vi "TriggerExample.vi"() -> ()   [LabVIEW 2016]
uses:
  controls/RunMode.ctl
  controls/TriggerNo.ctl
panel:
  out "Numeric":i32
  out "Message":string
  out "data out 2":string
  out "ExecConNo":i32
  out "RegisteredString":string
  out "ProgramNumber":i32
  out "SDCard":u16
  out "RunMode":T1
  out "error out":errorcluster
  out "data out":string
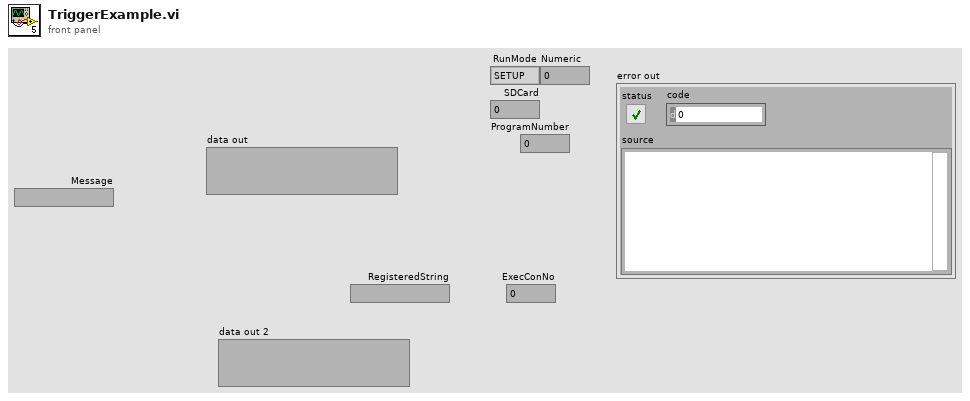
[diagram p1: front panel]
types:
  T1 = typedef "RunMode.ctl" = enum16{"SETUP", "RUN"}
  T2 = enum16{"Standard", "Buffered", "CRLF", "Immediate"}
  T3 = typedef "TriggerNo.ctl" = u8
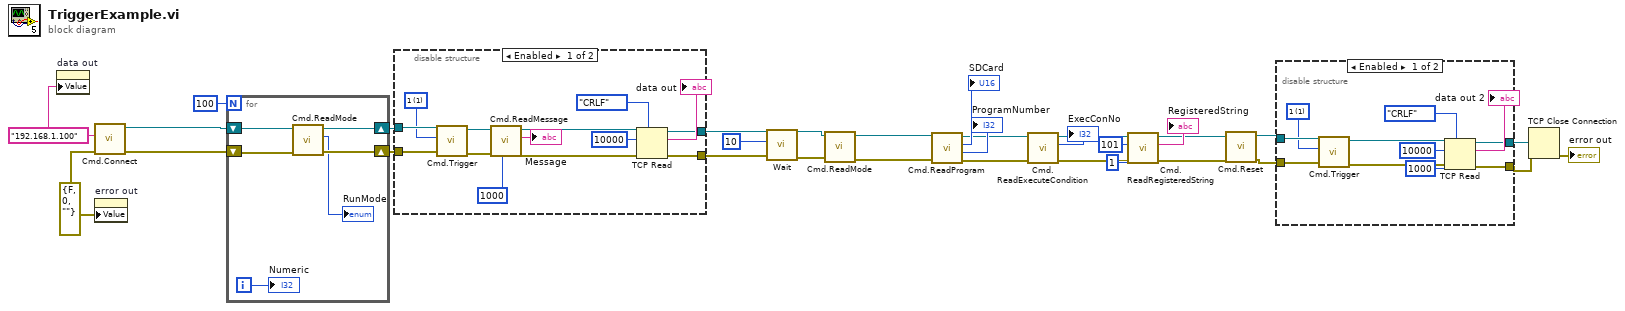
[diagram p0: block diagram]
diagram:
  w22 = errorcluster {"status"=FALSE, "code"=0, "source"=""} ("error constant")
  w21 = "192.168.1.100"
  n1 = property on="data out" class="Str"("Value"=w21) -> ()  [unwired: 2 in, 2 out]
  n2 = call "Cmd.Connect.vi"("error in (no error)"=w22, "IP"=w21) -> ("error out"=w2:errorcluster, "connection ID out"=w5:refnum<k5>)  [unwired: 8 in]
  n3 = property on="error out" class="Clust (strict)"("Value"=w22) -> ()  [unwired: 2 in, 2 out]
  n4 = for {
    N: 100 -> [_]
    shift-right: [w35] -> w4
    shift-left: w5 -> [w36]
    shift-right: [w34] -> w3
    shift-left: w2 -> [w33]
    i -> [w31]
    n5 = call "Cmd.ReadMode.vi"("error in"=w33, "cID in"=w36) -> ("error out"=w34:errorcluster, "RunMode"=→"RunMode":T1, "cID out"=w35:refnum<k5>)  [unwired: 7 in]
    "Numeric" <- w31
  }
  n6 = disable-structure shown="Enabled" {
    disable-tunnel: w4 -> [w50 w51]
    disable-tunnel: w3 -> [w49 w52]
    disable-tunnel: [w45 w52] -> w20
    disable-tunnel: [w44 w51] -> w17
    frame Enabled {
      w43 = T3 1 items=["1"=1, "2"=2, "3"=3, "4"=4, "ALL"=5] ("TriggerNo")
      n7 = call "Cmd.Trigger.vi"("error in"=w49, "TriggerNo"=w43, "cID in"=w50) -> ("error out"=w41:errorcluster, "cID out"=w42:refnum<k5>)  [unwired: 6 in, 1 out]
      n8 = call "Cmd.ReadMessage.vi"("Timeout [ms] (1000)"=1000 ("timeout ms (25000)"), "error in"=w41, "cID in"=w42) -> ("error out"=w39:errorcluster, "Message"=→"Message":string, "cID out"=w40:refnum<k5>)  [unwired: 6 in]
      n9 = TCP Read(connection ID=w40, bytes to read=10000, error in (no error)=w39, 7:T2."CRLF" ("mode (standard)")) -> (connection ID out=w44:refnum<k5>, data out=→"data out":string, error out=w45:errorcluster)  [unwired: 1 in]
    }
    frame Disabled {
    }
  }
  n10 = call "Wait.vi"("error in (no error)"=w20, "Time(ms)"=10) -> ("error out"=w19:errorcluster)  [unwired: 9 in]
  n11 = call "Cmd.ReadMode.vi"("error in"=w19, "cID in"=w17) -> ("error out"=w28:errorcluster, "cID out"=w29:refnum<k5>)  [unwired: 7 in, 1 out]
  n12 = call "Cmd.ReadProgram.vi"("error in"=w28, "cID in"=w29) -> ("error out"=w15:errorcluster, "ProgramNumber"=→"ProgramNumber":u16, "SDCard"=→"SDCard":u8, "cID out"=w16:refnum<k5>)  [unwired: 6 in]
  n13 = call "Cmd.ReadExecuteCondition.vi"("error in"=w15, "cID in"=w16) -> ("error out"=w13:errorcluster, "ExecConNo"=→"ExecConNo":i32, "cID out"=w14:refnum<k5>)  [unwired: 7 in]
  n14 = call "Cmd.ReadRegisteredString.Vi"("error in"=w13, "LineNo"=u8 1, "ToolNo"=u16 101, "cID in"=w14) -> ("error out"=w11:errorcluster, "RegisteredString"=→"RegisteredString":string, "cID out"=w10:refnum<k5>)  [unwired: 5 in]
  n15 = call "Cmd.Reset.vi"("error in"=w11, "cID in"=w10) -> ("error out"=w6:errorcluster, "cID out"=w9:refnum<k5>)  [unwired: 8 in]
  n16 = disable-structure shown="Enabled" {
    disable-tunnel: w9 -> [w63 w64]
    disable-tunnel: w6 -> [w62 w65]
    disable-tunnel: [w55 w65] -> w7
    disable-tunnel: [w54 w64] -> w8
    frame Enabled {
      w53 = T3 1 items=["1"=1, "2"=2, "3"=3, "4"=4, "ALL"=5] ("TriggerNo")
      n17 = call "Cmd.Trigger.vi"("error in"=w62, "TriggerNo"=w53, "cID in"=w63) -> ("error out"=w60:errorcluster, "cID out"=w61:refnum<k5>)  [unwired: 6 in, 1 out]
      n18 = TCP Read(connection ID=w61, bytes to read=10000, error in (no error)=w60, 7:T2."CRLF" ("mode (standard)"), 9:1000 ("timeout ms (25000)")) -> (connection ID out=w54:refnum<k5>, data out=→"data out 2":string, error out=w55:errorcluster)
    }
    frame Disabled {
    }
  }
  n19 = TCP Close Connection(connection ID=w8, error in (no error)=w7) -> (error out=→"error out":errorcluster)  [unwired: 1 in, 1 out]
